vi "Read Configuration.vi"(8 "error in":errorcluster) -> (0 "error out":errorcluster, 3 "Configuration":T1)   [LabVIEW 2020]
uses:
  <vilib>/Utility/config.llb/NI_LVConfig.lvlib
  Configuration--cluster.ctl
  <vilib>/Utility/config.llb/Read Key (String).vi
  <vilib>/Utility/config.llb/Read Key (Boolean).vi
  <vilib>/Utility/config.llb/Read Key (I32).vi
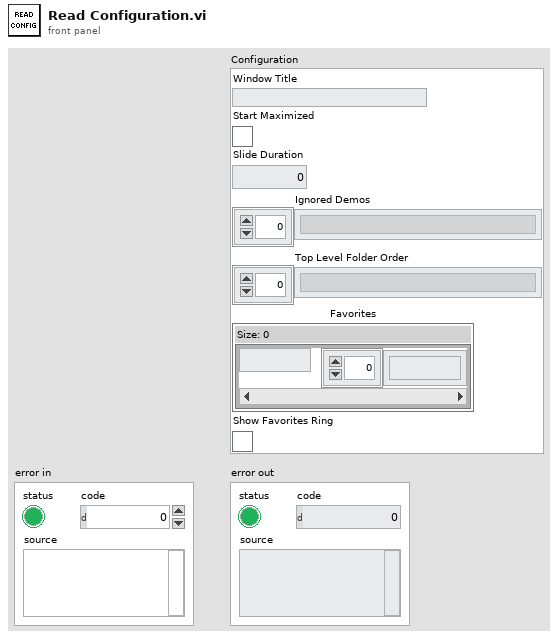
[diagram p1: front panel]
types:
  T1 = typedef "Configuration--cluster.ctl" = cluster{"Window Title":string, "Start Maximized":bool, "Slide Duration":i32, "Ignored Demos":string[], "Top Level Folder Order":string[], "Favorites":map{string, string[]}, "Show Favorites Ring":bool}
  T2 = typedef "NI_LVConfig.lvlib/Config Data RefNum.ctl" = refnum<k1>
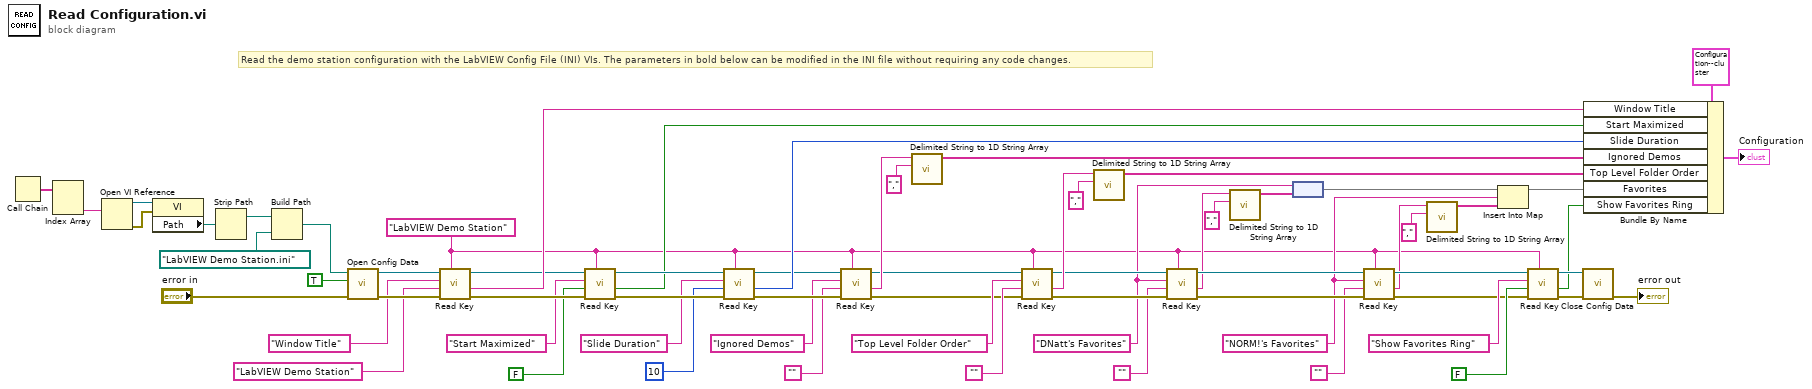
[diagram p0: block diagram]
diagram:
  w22 = "NORM!'s Favorites" ("key")
  w28 = "DNatt's Favorites" ("key")
  w2 = "LabVIEW Demo Station" ("section")
  # "Read the demo station configuration with the LabVIEW Config File (INI) VIs. The parameters in bold below can be modified in the INI file without requiring any code changes."
  n1 = Call Chain() -> (call chain=w20:string[])
  n2 = Index Array(array=w20) -> (element #2=w19:string)  [unwired: 2 in, 1 out]
  n3 = Open VI Reference(vi path=w19) -> (vi reference=w18:refnum<vi>, error out=w16:errorcluster)  [unwired: 5 in]
  n4 = property class="VI"(reference=w18, error in=w16) -> ("Path"=w17:path)  [unwired: 2 out]
  n5 = Strip Path(path=w17) -> (stripped path=w15:path)  [unwired: 1 out]
  n6 = Build Path(base path=w15, name or relative path=path "LabVIEW Demo Station.ini") -> (appended path=w64:path)
  n7 = call <vilib>:"Open Config Data.vi"("error in (no error)"="error in", "create file if necessary (T)"=TRUE, "configuration file path"=w64) -> ("error out"=w61:errorcluster, "refnum"=w60:T2)  [unwired: 6 in, 1 out]
  n8 = call-poly <vilib>:"Read Key.vi"("section"=w2, "error in (no error)"=w61, "default value"="LabVIEW Demo Station" ("section"), "key"="Window Title", "refnum"=w60) -> ("error out"=w55:errorcluster, "value"=w56:string, "refnum out"=w54:T2)  [unwired: 3 in, 1 out]
  n9 = call-poly <vilib>:"Read Key.vi"("section"=w2, "error in (no error)"=w55, "default value"=FALSE, "key"="Start Maximized", "refnum"=w54) -> ("error out"=w51:errorcluster, "value"=w48:bool, "refnum out"=w50:T2)  [unwired: 3 in, 1 out]
  n10 = call-poly <vilib>:"Read Key.vi"("section"=w2, "error in (no error)"=w51, "default value"=10, "key"="Slide Duration", "refnum"=w50) -> ("error out"=w44:errorcluster, "value"=w45:i32, "refnum out"=w43:T2)  [unwired: 3 in, 1 out]
  n11 = call-poly <vilib>:"Read Key.vi"("section"=w2, "error in (no error)"=w44, "default value"="", "key"="Ignored Demos", "refnum"=w43) -> ("error out"=w32:errorcluster, "value"=w41:string, "refnum out"=w33:T2)  [unwired: 3 in, 1 out]
  n12 = call <vilib>:"Delimited String to 1D String Array.vi"("delimiter"=",", "delimited string"=w41) -> ("string array"=w40:string[])  [unwired: 9 in]
  n13 = call-poly <vilib>:"Read Key.vi"("section"=w2, "error in (no error)"=w32, "default value"="", "key"="Top Level Folder Order", "refnum"=w33) -> ("error out"=w30:errorcluster, "value"=w35:string, "refnum out"=w29:T2)  [unwired: 3 in, 1 out]
  n14 = call <vilib>:"Delimited String to 1D String Array.vi"("delimiter"=",", "delimited string"=w35) -> ("string array"=w31:string[])  [unwired: 9 in]
  n15 = call-poly <vilib>:"Read Key.vi"("section"=w2, "error in (no error)"=w30, "default value"="", "key"=w28, "refnum"=w29) -> ("error out"=w24:errorcluster, "value"=w6:string, "refnum out"=w25:T2)  [unwired: 3 in, 1 out]
  n16 = call <vilib>:"Delimited String to 1D String Array.vi"("delimiter"=",", "delimited string"=w6) -> ("string array"=w27:string[])  [unwired: 9 in]
  n17 = node(w28, w27) -> (w26:map{string, string[]})
  n18 = call-poly <vilib>:"Read Key.vi"("section"=w2, "error in (no error)"=w24, "default value"="", "key"=w22, "refnum"=w25) -> ("error out"=w12:errorcluster, "value"=w3:string, "refnum out"=w9:T2)  [unwired: 3 in, 1 out]
  n19 = call <vilib>:"Delimited String to 1D String Array.vi"("delimiter"=",", "delimited string"=w3) -> ("string array"=w21:string[])  [unwired: 9 in]
  n20 = Insert Into Map(map in=w26, key=w22, value=w21) -> (map out=w23:map{string, string[]})  [unwired: 2 out]
  n21 = call-poly <vilib>:"Read Key.vi"("section"=w2, "error in (no error)"=w12, "default value"=FALSE, "key"="Show Favorites Ring", "refnum"=w9) -> ("error out"=w11:errorcluster, "value"=w1:bool, "refnum out"=w10:T2)  [unwired: 3 in, 1 out]
  n22 = call <vilib>:"Close Config Data.vi"("error in (no error)"=w11, "refnum"=w10) -> ("error out"=→"error out":errorcluster)  [unwired: 8 in, 1 out]
  n23 = Bundle By Name(cluster=T1 {"Window Title"="", "Start Maximized"=FALSE, "Slide Duration"=0, "Ignored Demos"=[], "Top Level Folder Order"=[], "Favorites"={}, "Show Favorites Ring"=FALSE} ("Configuration"), "Window Title"=w56, "Start Maximized"=w48, "Slide Duration"=w45, "Ignored Demos"=w40, "Top Level Folder Order"=w31, "Favorites"=w23, "Show Favorites Ring"=w1) -> (→"Configuration":T1)
